vi "GetFieldFromProtobufIndexGreeter_res_res_oneof.vi"(1 "protobuf index":i32) -> (0 "oneof field name":string)   [LabVIEW 2019, in "Generated_server.lvlib" / "Greeter_res_res_oneof.lvclass"]
uses:
  Greeter_res_res_oneof.lvclass
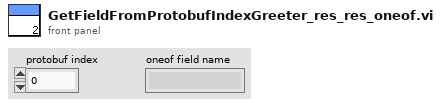
[diagram p1: front panel]
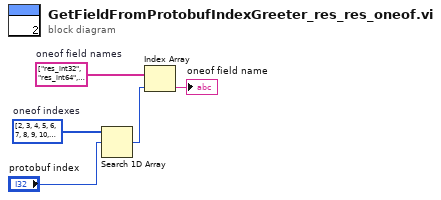
[diagram p0: block diagram]
diagram:
  w5 = string[] ["res_int32", "res_int64", "res_uint32", "res_uint64", "res_sint32", "res_sint64", "res_fixed32", "res_fixed64", "res_sfixed32", "res_sfixed64", "res_float", "res_double", "res_bool", "res_string", "res_bytes", "res_int32", "res_int64", "res_uint32", "res_uint64", "res_sint32", "res_sint64", "res_fixed32", "res_fixed64", "res_sfixed32", "res_sfixed64", "res_float", "res_double", "res_bool", "res_string", "res_bytes"]  # oneof field names
  w4 = i32[] [2, 3, 4, 5, 6, 7, 8, 9, 10, 11, 12, 13, 14, 15, 16, 2, 3, 4, 5, 6, 7, 8, 9, 10, 11, 12, 13, 14, 15, 16]  # oneof indexes
  n1 = Search 1D Array(1D array=w4, element="protobuf index") -> (index of element=w2:i32)  [unwired: 1 in]
  n2 = Index Array(array=w5, index=w2) -> (element=→"oneof field name":string)
